vi "repositoryConfigurator Main.vi"() -> ()   [LabVIEW 2013]
doc: "This template is for the Queued Message Handler design pattern.\n\nThe Event Handling Loop generates messages based on user interface actions.\n\nThe Message Handling Loop processes messages generated by the Event Handling Loop, or by other messages. The messages are string values, so new messages can be added easily to the Message Cases case structure in the Message Handling Loop. Each message cluster can also provide an optional value for Message Data, which is a variant that can be converted to whatever message-specific data is required."
uses:
  controls/repositoryConfigurator UI Data.ctl
  repoHandler/repoHandler.lvclass
  support/Message Queue/Enqueue Message (Single).vi
  <vilib>/Utility/error.llb/Error Cluster From Error Code.vi
  support/Message Queue/Enqueue Message (Array).vi
  <vilib>/ErrorRing/Error Ring.xnode
  support/Message Queue/repositoryConfigurator Message Queue.lvlib
  support/User Event - Stop/repositoryConfigurator User Event - Stop.lvlib
panel:
  out "Data":T1
  out "i":i32
  out "i2":i32
  in  "Apply":bool
  out "Log":string
  in  "Configuration file":path
  out "Repositories":string[][](table)
  in  "Save":bool
  in  "Refresh":bool
  in  "Exit":bool
  # "Server/Local mismatch\nNo server conn.\nOK"
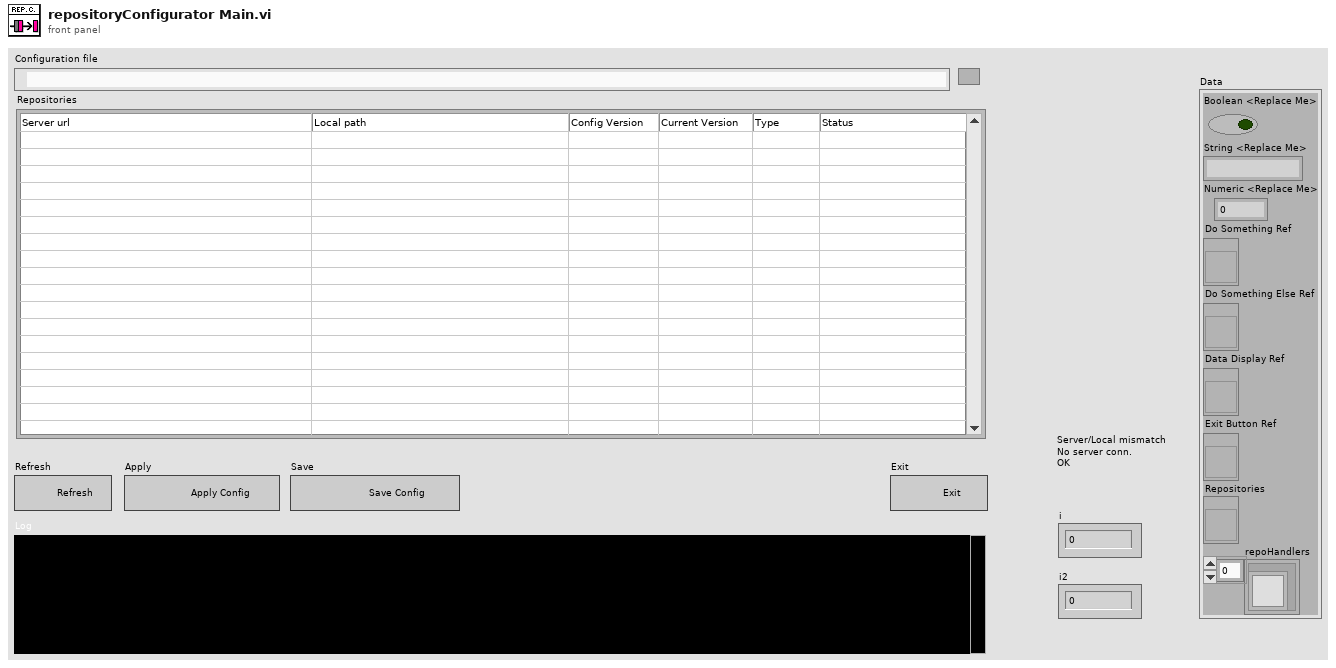
[diagram p1: front panel]
types:
  T1 = typedef "repositoryConfigurator UI Data.ctl" = cluster{"Boolean <Replace Me>":bool, "String <Replace Me>":string, "Numeric <Replace Me>":dbl, "Do Something Ref":refnum<vi>, "Do Something Else Ref":refnum<vi>, "Data Display Ref":refnum<vi>, "Exit Button Ref":refnum<vi>, "Repositories":refnum<vi>, "repoHandlers":refnum<class "repoHandler.lvclass">[]}
  T2 = typedef "repositoryConfigurator Message Queue.lvlib/All Message Queues.ctl" = cluster{"Repository":refnum<queue>, "log":refnum<queue>, "events":refnum<queue>}
  T3 = typedef "LVPoint32TypeDef.ctl" = cluster{"Horizontal":i32, "Vertical":i32}
  T4 = typedef "LVRowAndColumnTypeDef.ctl" = cluster{"Row":i32, "Column":i32}
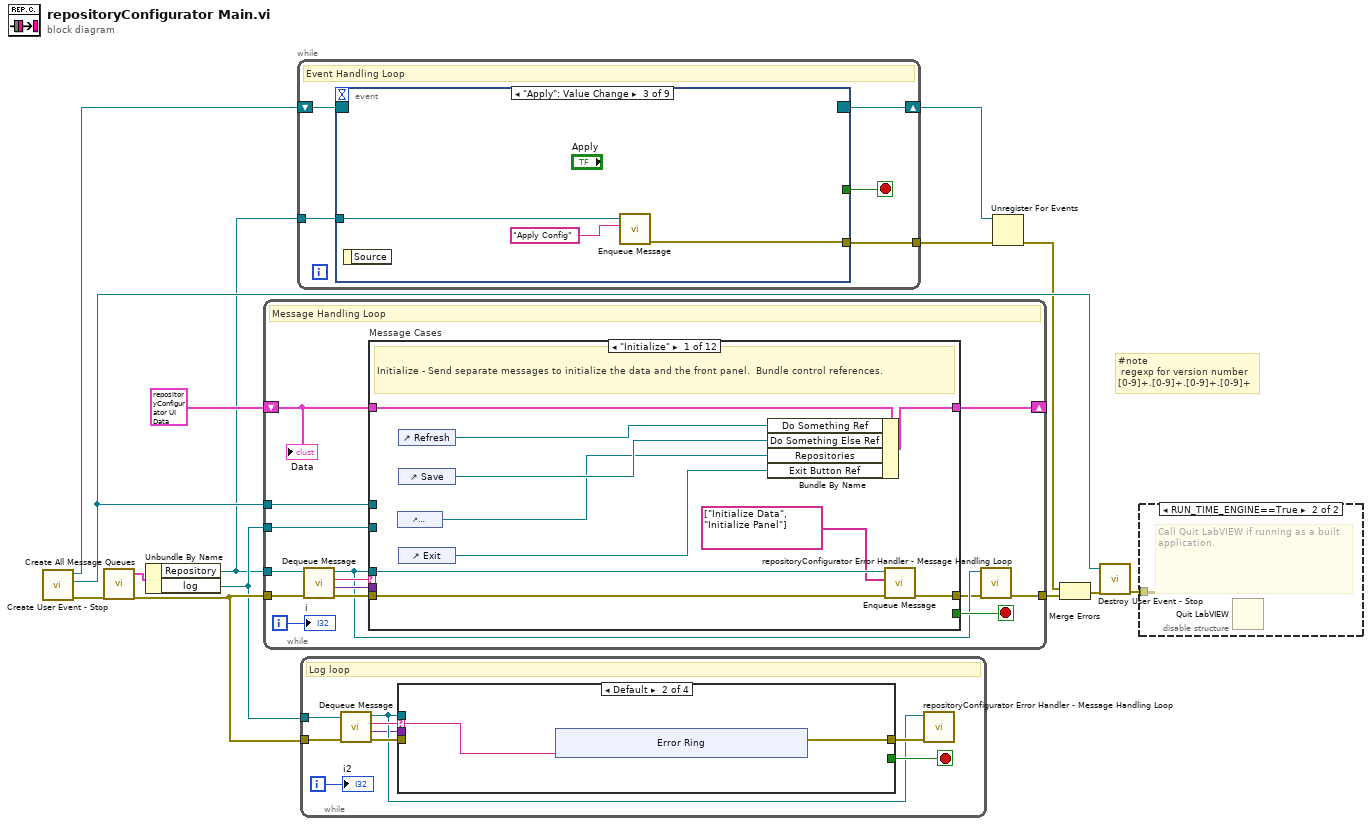
[diagram p0: block diagram]
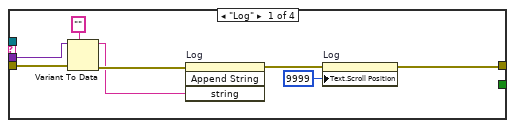
[diagram p2: hidden frame]
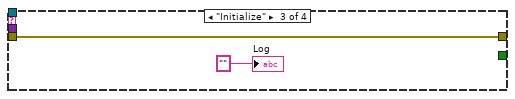
[diagram p3: hidden frame]
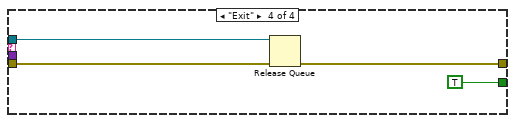
[diagram p4: hidden frame]
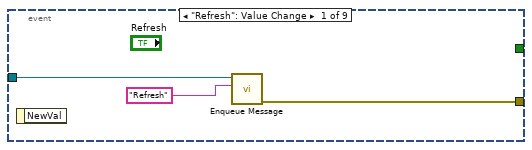
[diagram p6: hidden frame]
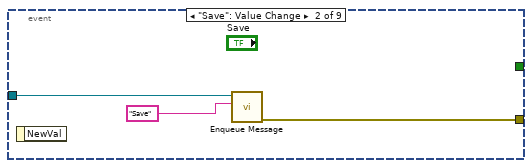
[diagram p7: hidden frame]
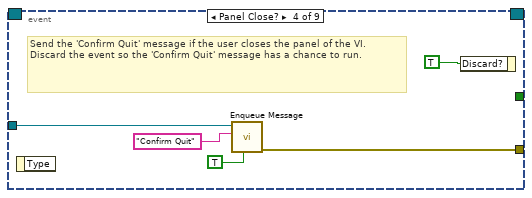
[diagram p8: hidden frame]
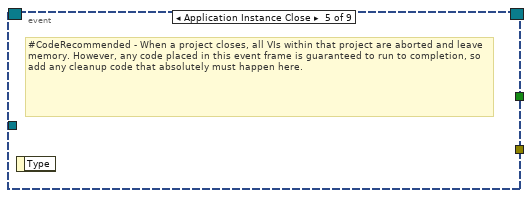
[diagram p9: hidden frame]
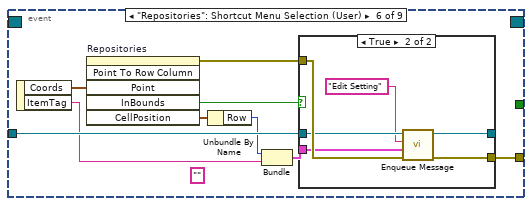
[diagram p10: hidden frame]
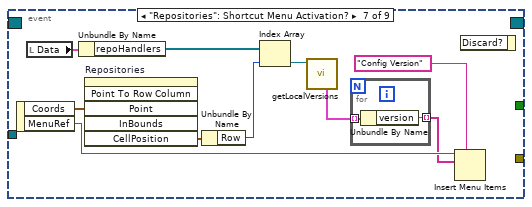
[diagram p12: hidden frame]
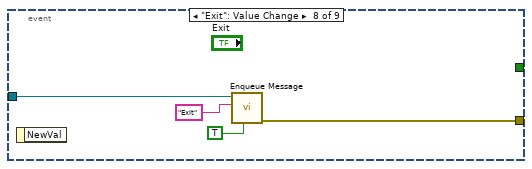
[diagram p13: hidden frame]
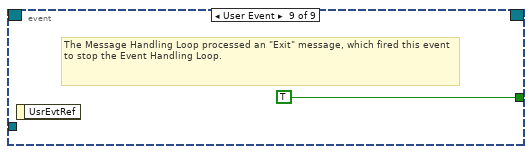
[diagram p14: hidden frame]
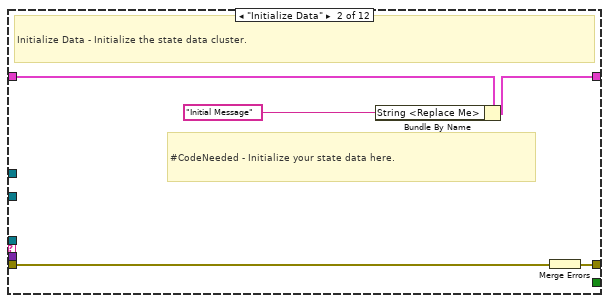
[diagram p15: hidden frame]
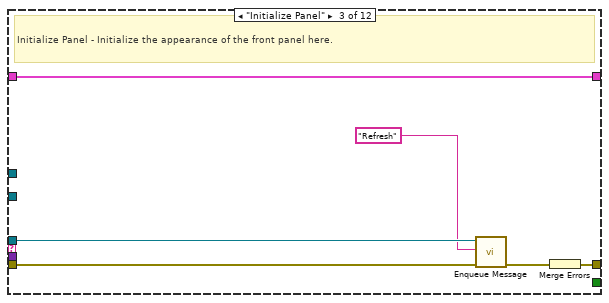
[diagram p16: hidden frame]
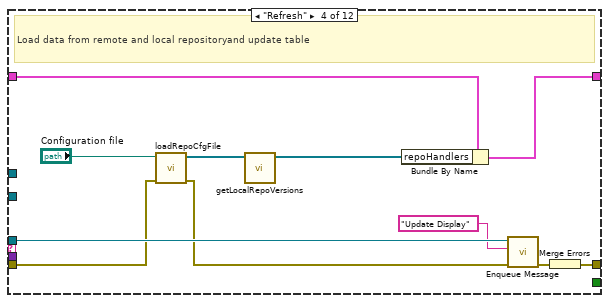
[diagram p17: hidden frame]
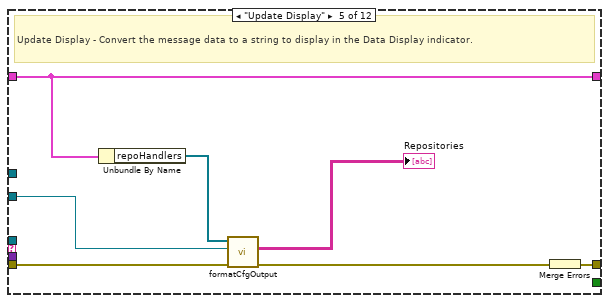
[diagram p18: hidden frame]
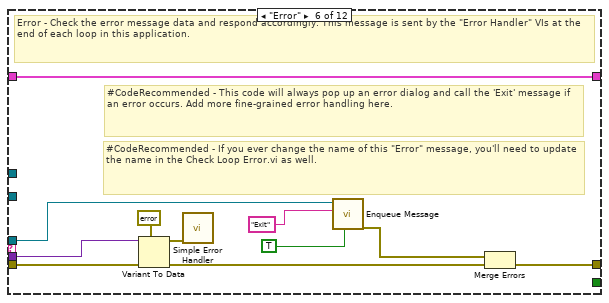
[diagram p19: hidden frame]
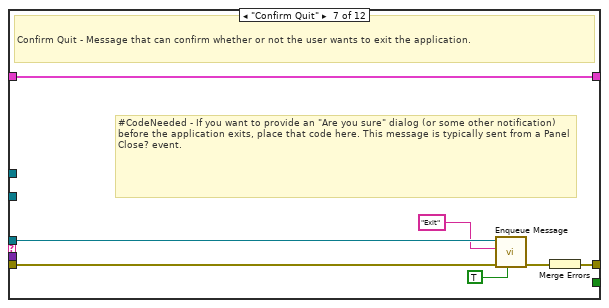
[diagram p20: hidden frame]
diagram:
  # "#note\n regexp for version number\n[0-9]+.[0-9]+.[0-9]+.[0-9]+"
  n1 = call "Create User Event - Stop.vi"() -> ("error out"=w11:errorcluster, "User Event - Stop"=w9:refnum<user-event>, "Stop Event Registration Refnum"=w12:refnum<event-registration>)  [unwired: 9 in]
  n2 = call "Create All Message Queues.vi"("error in (no error)"=w11) -> ("error out"=w3:errorcluster, "Message Queues out"=w14:T2)  [unwired: 9 in]
  n3 = Unbundle By Name(w14) -> ("Repository"=w1:refnum<queue>, "log"=w2:refnum<queue>)
  n4 = while {
    tunnel: w1 -> [w20]
    shift-right: [w27] -> _
    shift-left: T1 {"Boolean <Replace Me>"=FALSE, "String <Replace Me>"="", "Numeric <Replace Me>"=0.0, "Do Something Ref"=refnum, "Do Something Else Ref"=refnum, "Data Display Ref"=refnum, "Exit Button Ref"=refnum, "Repositories"=refnum, "repoHandlers"=[]} ("Data Cluster") -> [w28]
    tunnel: w9 -> [w25]
    tunnel: w3 -> [w24]
    tunnel: [w18] -> w13
    tunnel: w2 -> [w16]
    i -> [w15]
    stop <- w26 stop-if-true
    # "Message Handling Loop"
    n5 = call "Dequeue Message.vi"("error in (no error)"=w24, "Message Queue"=w20) -> ("error out"=w23:errorcluster, "Message Data"=w21:variant, "Message"=w22:string, "dup Message Queue"=w19:refnum<queue>)  [unwired: 6 in]
    n6 = case "Message Cases" shown="\"Initialize\"" w22 {
      selector: w22 -> [_ _ _ _ _ _ _ _ _ _ _ w178]
      tunnel: w19 -> [w36 _ w46 w58 _ w70 w81 _ w90 w120 w177 _]
      tunnel: w23 -> [w37 w43 w47 w55 w65 w78 w85 w88 w97 w129 w172 _]
      tunnel: [w38 w39 w48 w60 w67 w71 w83 w86 w96 w130 w173 w179] -> w17
      tunnel: w28 -> [w35 w42 w49 w54 w63 w77 w84 w87 w93 w123 w176 w180]
      tunnel: [w34 w41 w49 w53 w63 w77 w84 w87 w92 w122 w176 w180] -> w27
      tunnel: [_ _ _ _ _ _ _ _ _ _ TRUE _] -> w26
      tunnel: w21 -> [_ _ _ _ _ w76 _ _ _ w128 _ _]
      tunnel: w25 -> [_ _ _ _ _ _ _ _ _ _ w171 _]
      tunnel: w16 -> [_ _ _ _ w61 _ _ _ w94 _ w170 _]
      frame "Initialize" {
        # "Initialize - Send separate messages to initialize the data and the front panel.  Bundle control references."
        n7 = control-ref of="Repositories"() -> (w29:refnum<vi>)
        n8 = control-ref of="Refresh"() -> (w33:refnum<vi>)
        n9 = control-ref of="Save"() -> (w32:refnum<vi>)
        n10 = control-ref of="Exit"() -> (w31:refnum<vi>)
        n11 = Bundle By Name(cluster=w35, "Do Something Ref"=w33, "Do Something Else Ref"=w32, "Repositories"=w29, "Exit Button Ref"=w31) -> (w34:T1)
        n12 = call-poly "Enqueue Message.vi"("error in (no error)"=w37, "Message Array"=string[] ["Initialize Data", "Initialize Panel"], "Message Queue"=w36) -> ("error out"=w38:errorcluster)  [unwired: 7 in, 1 out]
      }
      frame "Initialize Data" {
        # "#CodeNeeded - Initialize your state data here."
        # "Initialize Data - Initialize the state data cluster."
        n13 = Bundle By Name(cluster=w42, "String <Replace Me>"="Initial Message" ("Initial Message")) -> (w41:T1)
        n14 = Merge Errors(w43) -> (w39:errorcluster)
      }
      frame "Initialize Panel" {
        # "Initialize Panel - Initialize the appearance of the front panel here."
        n15 = call-poly "Enqueue Message.vi"("error in (no error)"=w47, "Message"="Refresh", "Message Queue"=w46) -> ("error out"=w45:errorcluster)  [unwired: 7 in, 1 out]
        n16 = Merge Errors(w45) -> (w48:errorcluster)
      }
      frame "Refresh" {
        # "Load data from remote and local repositoryand update table"
        n17 = call "loadRepoCfgFile.vi"("error in (no error)"=w55, "path to XML document"="Configuration file") -> ("error out"=w51:errorcluster, "repoHandlers"=w52:refnum<class "repoHandler.lvclass">[])  [unwired: 8 in]
        n18 = call "getLocalRepoVersions.vi"("repoHandlers in"=w52) -> ("repoHandlers"=w50:refnum<class "repoHandler.lvclass">[])  [unwired: 9 in, 1 out]
        n19 = Bundle By Name(cluster=w54, "repoHandlers"=w50) -> (w53:T1)
        n20 = call-poly "Enqueue Message.vi"("error in (no error)"=w51, "Message"="Update Display", "Message Queue"=w58) -> ("error out"=w59:errorcluster)  [unwired: 7 in, 1 out]
        n21 = Merge Errors(w59) -> (w60:errorcluster)
      }
      frame "Update Display" {
        # "Update Display - Convert the message data to a string to display in the Data Display indicator."
        n22 = Unbundle By Name(w63) -> ("repoHandlers"=w62:refnum<class "repoHandler.lvclass">[])
        n23 = call "formatCfgOutput.vi"("error in (no error)"=w65, "Log Message Queue"=w61, "repoHandlers"=w62) -> ("error out"=w64:errorcluster, "tableOutput"=→"Repositories":string[][])  [unwired: 6 in, 1 out]
        n24 = Merge Errors(w64) -> (w67:errorcluster)
      }
      frame "Error" {
        # "#CodeRecommended - If you ever change the name of this \"Error\" message, you'll need to update the name in the Check Loop Error.vi as well."
        # "#CodeRecommended - This code will always pop up an error dialog and call the 'Exit' message if an error occurs. Add more fine-grained error handling here."
        # "Error - Check the error message data and respond accordingly. This message is sent by the \"Error Handler\" VIs at the end of each loop in this application."
        n25 = Variant To Data(error in=w78, type=errorcluster {"status"=FALSE, "code"=0, "source"=""} ("error constant"), Variant=w76) -> (data=w74:errorcluster, error out=w73:errorcluster)
        n26 = call <vilib>:"Simple Error Handler.vi"("error in (no error)"=w74) -> ()  [unwired: 4 in, 5 out]
        n27 = call-poly "Enqueue Message.vi"("Priority Message? (F)"=TRUE, "Message"="Exit", "Message Queue"=w70) -> ("error out"=w72:errorcluster)  [unwired: 7 in, 1 out]
        n28 = Merge Errors(w72, w73) -> (w71:errorcluster)
      }
      frame "Confirm Quit" {
        # "#CodeNeeded - If you want to provide an \"Are you sure\" dialog (or some other notification) before the application exits, place that code here. This message is typically sent from a Panel Close? event."
        # "Confirm Quit - Message that can confirm whether or not the user wants to exit the application."
        n29 = call-poly "Enqueue Message.vi"("Priority Message? (F)"=TRUE, "error in (no error)"=w85, "Message"="Exit", "Message Queue"=w81) -> ("error out"=w82:errorcluster)  [unwired: 6 in, 1 out]
        n30 = Merge Errors(w82) -> (w83:errorcluster)
      }
      frame "---Copy This Frame---" {
        # "Duplicate this frame when creating new messages.  Change this comment in the duplicated frame to describe this message."
        n31 = Merge Errors(w88) -> (w86:errorcluster)
      }
      frame "Apply Config" {
        # "Duplicate this frame when creating new messages.  Change this comment in the duplicated frame to describe this message."
        n32 = Unbundle By Name(w93) -> ("repoHandlers"=w95:refnum<class "repoHandler.lvclass">[])
        n33 = for {
          tunnel: w95 -> [w114] mode=indexing
          tunnel: w94 -> [w109]
          tunnel: [w107] -> w91 mode=indexing
          tunnel: ["Update Display" ("Message")] -> w89
          n34 = call-dynamic "getConfigVersion.vi"("repoHandler in"=w114) -> ("error out"=w111:errorcluster, "repoHandler out"=w113:refnum<class "repoHandler.lvclass">, "Config Version"=w112:string)  [unwired: 8 in]
          n35 = call-dynamic "updateToVersion.vi"("error in (no error)"=w111, "Version"=w112, "repoHandler in"=w113) -> ("error out"=w104:errorcluster, "Log"=w108:string, "repoHandler out"=w106:refnum<class "repoHandler.lvclass">)  [unwired: 6 in]
          n36 = call-poly "Enqueue Message.vi"("Message Data"=w108, "Message"="Log", "Message Queue"=w109) -> ("dup Message Queue"=w100:refnum<queue>)  [unwired: 7 in, 1 out]
          n37 = call-dynamic "getCurrentVersion.vi"("error in (no error)"=w104, "repoHandler in"=w106) -> ("error out"=w103:errorcluster, "Log"=w101:string, "repoHandler out"=w105:refnum<class "repoHandler.lvclass">, "Local Version"=w99:string)  [unwired: 6 in]
          n38 = call-poly "Enqueue Message.vi"("Message Data"=w101, "Message"="Log", "Message Queue"=w100) -> ()  [unwired: 7 in, 2 out]
          n39 = call-dynamic "setCurrentVersion.vi"("error in (no error)"=w103, "Current Version"=w99, "repoHandler in"=w105) -> ("repoHandler out"=w107:refnum<class "repoHandler.lvclass">)  [unwired: 7 in, 1 out]
        }
        n40 = Bundle By Name(cluster=w93, "repoHandlers"=w91) -> (w92:T1)
        n41 = Merge Errors(w97) -> (w96:errorcluster)
        n42 = call-poly "Enqueue Message.vi"("Message"=w89, "Message Queue"=w90) -> ()  [unwired: 8 in, 2 out]
      }
      frame "Edit Setting" {
        # "Edit Server URL"
        n43 = Unbundle By Name(w123) -> ("repoHandlers"=w125:refnum<class "repoHandler.lvclass">[])
        n44 = Variant To Data(error in=w129, type=cluster{"Row":i32, "ItemTag":string} {"Row"=0, "ItemTag"=""} ("cluster"), Variant=w128) -> (data=w118:cluster{"Row":i32, "ItemTag":string}, error out=w121:errorcluster)
        n45 = Unbundle By Name(w118) -> ("Row"=w116:i32, "ItemTag"=w117:string)
        n46 = in-place {
          in-place-border: w121 -> [w132]
          in-place-border: w117 -> [w133]
          in-place-border: [w131] -> w115
          n47 = in-place-array #1(w125, w116) -> (w135:refnum<class "repoHandler.lvclass">)
          n48 = case shown="\"Config Version\"" w133 {
            selector: w133 -> [w138 _ _ _ _]
            tunnel: w135 -> [w140 w142 w147 w154 w162]
            tunnel: [w139 w142 w146 w153 w161] -> w134
            tunnel: w132 -> [w137 w141 w144 w152 w160]
            tunnel: [w136 w141 w143 w151 w159] -> w131
            frame Default {
              n49 = call-dynamic "setVersion.vi"("error in (no error)"=w137, "setVersion"=w138, "repoHandler in"=w140) -> ("error out"=w136:errorcluster, "repoHandler out"=w139:refnum<class "repoHandler.lvclass">)  [unwired: 7 in]
            }
            frame "Config Version" {
            }
            frame "Edit Type" {
              n50 = call-dynamic "getType.vi"("error in (no error)"=w144, "repoHandler in"=w147) -> ("error out"=w150:errorcluster, "repoHandler out"=w148:refnum<class "repoHandler.lvclass">, "Type"=w145:string)  [unwired: 7 in]
              n51 = call "inputPopup.vi"("default text"=w145) -> ("value"=w149:string)  [unwired: 10 in]
              n52 = call-dynamic "setType.vi"("error in (no error)"=w150, "Type"=w149, "repoHandler in"=w148) -> ("error out"=w143:errorcluster, "repoHandler out"=w146:refnum<class "repoHandler.lvclass">)  [unwired: 7 in]
            }
            frame "Edit Local Path" {
              n53 = call-dynamic "getLocalPath.vi"("error in (no error)"=w152, "repoHandler in"=w154) -> ("error out"=w158:errorcluster, "repoHandler out"=w156:refnum<class "repoHandler.lvclass">, "Local Path"=w157:string)  [unwired: 7 in]
              n54 = call "inputPopup.vi"("default text"=w157) -> ("value"=w155:string)  [unwired: 10 in]
              n55 = call-dynamic "setLocalPath.vi"("error in (no error)"=w158, "localPath"=w155, "repoHandler in"=w156) -> ("error out"=w151:errorcluster, "repoHandler out"=w153:refnum<class "repoHandler.lvclass">)  [unwired: 7 in]
            }
            frame "Edit Server URL" {
              n56 = call-dynamic "getServerUrl.vi"("error in (no error)"=w160, "repoHandler in"=w162) -> ("error out"=w163:errorcluster, "repoHandler out"=w165:refnum<class "repoHandler.lvclass">, "Server url"=w166:string)  [unwired: 7 in]
              n57 = call "inputPopup.vi"("default text"=w166) -> ("value"=w164:string)  [unwired: 10 in]
              n58 = call-dynamic "setServerUrl.vi"("error in (no error)"=w163, "serverUrl"=w164, "repoHandler in"=w165) -> ("error out"=w159:errorcluster, "repoHandler out"=w161:refnum<class "repoHandler.lvclass">)  [unwired: 7 in]
            }
          }
          n59 = in-place-array #1(w134) -> (w124:refnum<class "repoHandler.lvclass">[])  [unwired: 1 out]
        }
        n60 = Bundle By Name(cluster=w123, "repoHandlers"=w124) -> (w122:T1)
        n61 = call-poly "Enqueue Message.vi"("error in (no error)"=w115, "Message"="Update Display", "Message Queue"=w120) -> ("error out"=w127:errorcluster)  [unwired: 7 in, 1 out]
        n62 = Merge Errors(w127) -> (w130:errorcluster)
      }
      frame "Exit" {
        # "Stop the VI"
        # "Release the message queue reference"
        # "Exit - Exit the application."
        n63 = Release Queue(queue=w177, error in (no error)=w172) -> (error out=w174:errorcluster)  [unwired: 1 in, 2 out]
        n64 = call-poly "Enqueue Message.vi"("Message"="Exit", "Message Queue"=w170) -> ("error out"=w168:errorcluster)  [unwired: 8 in, 1 out]
        n65 = call "Fire User Event - Stop.vi"("User Event - Stop"=w171) -> ("error out"=w169:errorcluster)  [unwired: 10 in]
        n66 = Merge Errors(w169, w168, w174) -> (w173:errorcluster)
      }
      frame Default {
        # "'Default' case only runs if there is a message that isn't defined in any of the other cases.  Output a programming error."
        n67 = xnode "Error Ring"("parameter 0"=w178) -> ("error out"=w179:errorcluster)
      }
    }
    n68 = call "repositoryConfigurator Error Handler - Message Handling Loop.vi"("error in (no error)"=w17, "Message Queue"=w19) -> ("dup error in"=w18:errorcluster)  [unwired: 8 in, 1 out]
    "i" <- w15
    "Data" <- w28
  }
  n69 = while {
    shift-right: [w191] -> w7
    shift-left: w12 -> [w192]
    tunnel: [w188] -> w4
    tunnel: w1 -> [w189]
    stop <- w190 stop-if-true
    # "Event Handling Loop"
    n70 = event shown="[2] \"Apply\": Value Change" {
      selector: w192 -> [_ _ _ _ _ _ _ _ _]
      dyn-events: [_ _ _ _ _ _ _ _ _] -> w191
      timeout: _ -> [_ _ _ _ _ _ _ _ _]
      tunnel: [_ _ _ _ _ _ _ _ TRUE ("Discard?")] -> w190
      tunnel: [w194 w197 w200 w205 _ w215 _ w239 _] -> w188
      tunnel: w189 -> [w193 w196 w199 w202 _ w211 _ w236 _]
      event "Refresh": Value Change {
        n71 = event-data() -> ()  [unwired: 1 in, 1 out]
        n72 = call-poly "Enqueue Message.vi"("Message"="Refresh", "Message Queue"=w193) -> ("error out"=w194:errorcluster)  [unwired: 8 in, 1 out]
      }
      event "Save": Value Change {
        n73 = event-data() -> ()  [unwired: 1 in, 1 out]
        n74 = call-poly "Enqueue Message.vi"("Message"="Save", "Message Queue"=w196) -> ("error out"=w197:errorcluster)  [unwired: 8 in, 1 out]
      }
      event "Apply": Value Change {
        n75 = event-data() -> ()  [unwired: 1 in, 1 out]
        n76 = call-poly "Enqueue Message.vi"("Message"="Apply Config", "Message Queue"=w199) -> ("error out"=w200:errorcluster)  [unwired: 8 in, 1 out]
      }
      event Panel Close? {
        # "Send the 'Confirm Quit' message if the user closes the panel of the VI. Discard the event so the 'Confirm Quit' message has a chance to run."
        n77 = event-data() -> ()  [unwired: 1 in, 1 out]
        n78 = call-poly "Enqueue Message.vi"("Priority Message? (F)"=TRUE, "Message"="Confirm Quit", "Message Queue"=w202) -> ("error out"=w205:errorcluster)  [unwired: 7 in, 1 out]
        n79 = event-data("Discard?"=TRUE) -> ()  [unwired: 1 in, 1 out]
      }
      event Application Instance Close {
        # "#CodeRecommended - When a project closes, all VIs within that project are aborted and leave memory. However, any code placed in this event frame is guaranteed to run to completion, so add any cleanup code that absolutely must happen here."
        n80 = event-data() -> ()  [unwired: 1 in, 1 out]
      }
      event "Repositories": Shortcut Menu Selection (User) {
        (unwired) ""
        n81 = event-data() -> ("Coords"=w214:T3, "ItemTag"=w210:string)  [unwired: 1 in]
        n82 = invoke on="Repositories" class="Tbl (strict)" method="Point To Row Column"("Point"=w214) -> (error out=w213:errorcluster, "InBounds"=w212:bool, "CellPosition"=w209:T4)  [unwired: 5 in, 3 out]
        n83 = Unbundle By Name(w209) -> ("Row"=w208:i32)
        n84 = Bundle("Row"=w208, "ItemTag"=w210) -> (w207:cluster{"Row":i32, "ItemTag":string})  [unwired: 1 in]
        n85 = case shown="True" w212 {
          tunnel: [w216 w223] -> _
          tunnel: [w217 w222] -> w215
          tunnel: w213 -> [w217 w221]
          tunnel: w211 -> [w216 w220]
          tunnel: w207 -> [_ w218]
          frame False {
          }
          frame True {
            n86 = call-poly "Enqueue Message.vi"("error in (no error)"=w221, "Message Data"=w218, "Message"="Edit Setting", "Message Queue"=w220) -> ("error out"=w222:errorcluster, "dup Message Queue"=w223:refnum<queue>)  [unwired: 6 in]
          }
        }
      }
      event "Repositories": Shortcut Menu Activation? {
        n87 = event-data() -> ("Coords"=w232:T3, "MenuRef"=w227:refnum<k9>)  [unwired: 1 in]
        n88 = local read "Data"() -> (w231:T1)
        n89 = Unbundle By Name(w231) -> ("repoHandlers"=w230:refnum<class "repoHandler.lvclass">[])
        n90 = invoke on="Repositories" class="Tbl (strict)" method="Point To Row Column"("Point"=w232) -> ("CellPosition"=w233:T4)  [unwired: 5 in, 5 out]
        n91 = Unbundle By Name(w233) -> ("Row"=w229:i32)
        n92 = Index Array(array=w230, index=w229) -> (element=w228:refnum<class "repoHandler.lvclass">)
        n93 = call-dynamic "getLocalVersions.vi"("repoHandler in"=w228) -> ("Local Versions"=w226:cluster{"version":string, "longHash":string}[])  [unwired: 8 in, 2 out]
        n94 = for {
          tunnel: w226 -> [w235] mode=indexing
          tunnel: [w234] -> w225 mode=indexing
          n95 = Unbundle By Name(w235) -> ("version"=w234:string)
        }
        n96 = Insert Menu Items(5:"Config Version" ("menu tag"), 8:w225, 9:w227) -> ()  [unwired: 3 in, 3 out]
        n97 = event-data() -> ()  [unwired: 2 in, 1 out]
      }
      event "Exit": Value Change {
        n98 = event-data() -> ()  [unwired: 1 in, 1 out]
        n99 = call-poly "Enqueue Message.vi"("Priority Message? (F)"=TRUE, "Message"="Exit", "Message Queue"=w236) -> ("error out"=w239:errorcluster)  [unwired: 7 in, 1 out]
      }
      event User Event {
        # "The Message Handling Loop processed an \"Exit\" message, which fired this event to stop the Event Handling Loop."
        n100 = event-data() -> ()  [unwired: 1 in, 1 out]
      }
    }
  }
  n101 = while {
    tunnel: w2 -> [w249]
    tunnel: w3 -> [w248]
    i -> [w242]
    stop <- w244 stop-if-true
    # "Log loop"
    n102 = call "Dequeue Message.vi"("error in (no error)"=w248, "Message Queue"=w249) -> ("error out"=w247:errorcluster, "Message Data"=w241:variant, "Message"=w246:string, "dup Message Queue"=w243:refnum<queue>)  [unwired: 6 in]
    n103 = case shown="Default" w246 {
      selector: w246 -> [_ w258 _ _]
      tunnel: w247 -> [w254 _ w267 w272]
      tunnel: [w256 w259 w267 w271] -> w245
      tunnel: [_ _ _ TRUE] -> w244
      tunnel: w243 -> [_ _ _ w270]
      tunnel: w241 -> [w251 _ _ _]
      frame "Log" {
        n104 = Variant To Data(error in=w254, type="", Variant=w251) -> (data=w250:string, error out=w253:errorcluster)
        n105 = invoke on="Log" class="Str" method="Append String"(error in=w253, "string"=w250) -> (error out=w257:errorcluster)  [unwired: 2 in, 3 out]
        n106 = property on="Log" class="Str"(error in=w257, "Text.Scroll Position"=u32 9999) -> (error out=w256:errorcluster)  [unwired: 1 in, 1 out]
      }
      frame Default {
        n107 = xnode "Error Ring"("parameter 0"=w258) -> ("error out"=w259:errorcluster)
      }
      frame "Initialize" {
        "Log" <- ""
      }
      frame "Exit" {
        n108 = Release Queue(queue=w270, error in (no error)=w272) -> (error out=w271:errorcluster)  [unwired: 1 in, 2 out]
      }
    }
    n109 = call "repositoryConfigurator Error Handler - Message Handling Loop.vi"("error in (no error)"=w245, "Message Queue"=w243) -> ()  [unwired: 8 in, 2 out]
    "i2" <- w242
  }
  n110 = Unregister For Events(event registration refnum=w7, error in=w4) -> (error out=w8:errorcluster)
  n111 = Merge Errors(w8, w13) -> (w10:errorcluster)
  n112 = call "Destroy User Event - Stop.vi"("error in (no error)"=w10, "User Event - Stop"=w9) -> ("error out"=w5:errorcluster)  [unwired: 9 in]
  n113 = disable-structure shown="RUN_TIME_ENGINE==True" {
    disable-tunnel: w5 -> [_ _]
    frame condition #0 (active) {
    }
    frame condition #1 {
      # "Call Quit LabVIEW if running as a built application."
      n114 = Quit LabVIEW() -> ()  [unwired: 1 in]
    }
  }
